vi "PXI-Enumerate DIO Boards.vi"(8 "error in (no error)":errorcluster) -> (0 "error out":errorcluster, 2 "Devices":tag[](array[tag]))   [LabVIEW 2020]
uses:
  <resource>/objmgr/daqmx.rc
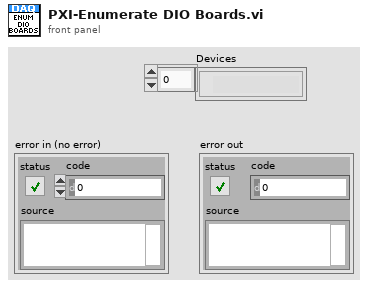
[diagram p1: front panel]
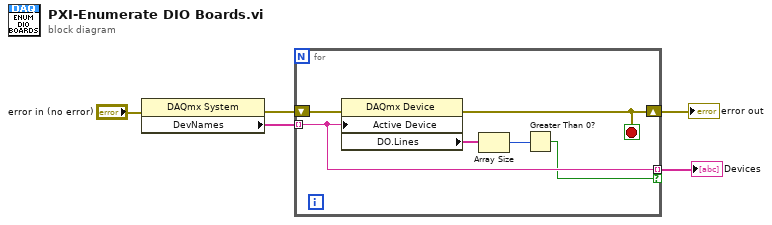
[diagram p0: block diagram]
diagram:
  n1 = property class="DAQmx System"(error in="error in (no error)") -> (error out=w5:errorcluster, "DevNames"=w4:tag[])  [unwired: 1 in, 1 out]
  n2 = for {
    tunnel: w4 -> [w7] mode=indexing
    shift-right: [w10] -> w2
    shift-left: w5 -> [w11]
    tunnel: [w7] -> w1 mode=indexing if=w6
    stop <- w10 stop-if-true
    n3 = property class="DAQmx Device"(error in=w11, "Active Device"=w7) -> (error out=w10:errorcluster, "DO.Lines"=w8:tag[])  [unwired: 1 in, 1 out]
    n4 = Array Size(array=w8) -> (size(s)=w9:i32)
    n5 = Greater Than 0?(x=w9) -> (x > 0?=w6:bool)
  }
  "error out" <- w2
  "Devices" <- w1
